vi "amp PID.vi"(0 "D gain":fxp<+/-,32,11>, 1 "Input":i16, 2 "hp coeff":i32[](array[numeric])=[946630756, 1010186290], 7 "I gain":fxp<+/-,32,11>, 8 "Upper limit":fxp<+/-,32,2>, 9 "P gain":fxp<+/-,32,11>, 10 "Lower limit":fxp<+/-,32,2>, 11 "Reset Integral":bool, 12 "DC offset":i16, 13 "lp coeff":i32[](array[numeric])=[1008310688, 32715568], 15 "final filter coeff":i32[](array[numeric])=[-955995012, 2025731616, 1001305, -1023351008, 2092954700, 1034533]) -> (3 "P gain check":fxp<+/-,32,2> format="%.31g", 4 "Final Filter check":fxp<+/-,32,2> format="%.31g", 5 "coerce check":fxp<+/-,32,2> format="%.31g", 6 "PID Output":fxp<+/-,32,2> format="%.26g", 14 "Divide check":fxp<+/-,32,2> format="%.31g")   [LabVIEW 2020]
uses:
  <vilib>/rvi/FXPMathLib/basic elements/FxpIntAccumulator/subVIs/nifxpmath_IntAccumulator_SimConfig.ctl
  <vilib>/rvi/FXPMathLib/basic elements/FxpIntAccumulator/simVIs/DllFxpIntAccumulator_sub.vi
  <vilib>/rvi/Analysis/measure/butterworth/XNode/niFpgaButterworthFilter.xnode
  <vilib>/rvi/FXPMathLib/basic elements/FxpIntAccumulator/XNode/nifxpmath_IntAccumulator.xnode
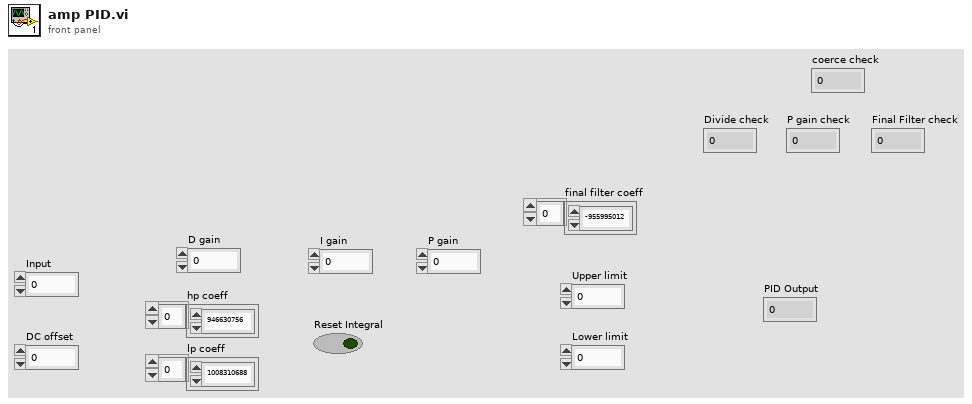
[diagram p1: front panel]
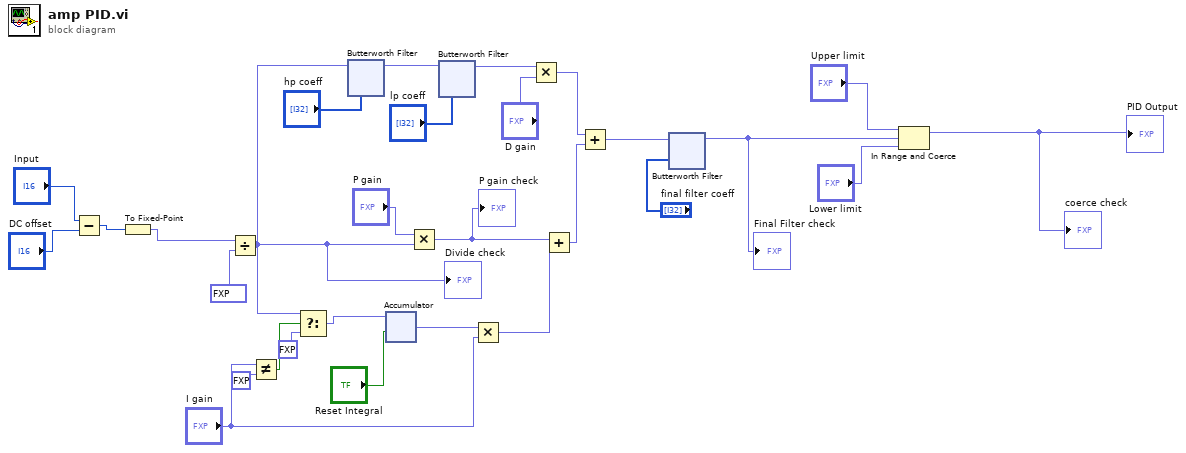
[diagram p0: block diagram]
diagram:
  n1 = Subtract(x="Input", y="DC offset") -> (x-y=w6:i16)
  n2 = To Fixed-Point(number=w6) -> (fixed-point=w5:fxp<+/-,32,16>)  [unwired: 1 in]
  n3 = Divide(x=w5, y=fxp<+,1,15> 16384.0) -> (x/y=w8:fxp<+/-,32,2>)
  "Divide check" <- w8
  n4 = Not Equal?(x="I gain", y=fxp<+/-,16,16> 0.0) -> (x != y?=w20:bool)
  n5 = Select(t=w8, s=w20, f=fxp<+/-,32,2> 0.0) -> (s? t:f=w18:fxp<+/-,32,2>)
  n6 = xnode "Butterworth Filter"("input data"=w8, "scaled coefficients"="hp coeff") -> ("output data"=w13:fxp<+/-,36,6>)  [unwired: 1 in]
  n7 = xnode "Accumulator"("x"=w18, "load (F)"="Reset Integral") -> ("s"=w29:fxp<+/-,46,16>)  [unwired: 3 in, 1 out]
  n8 = Multiply(x="P gain", y=w8) -> (x*y=w7:fxp<+/-,32,2>)
  "P gain check" <- w7
  n9 = xnode "Butterworth Filter"("input data"=w13, "scaled coefficients"="lp coeff") -> ("output data"=w12:fxp<+/-,36,10>)  [unwired: 1 in]
  n10 = Multiply(x=w29, y="I gain") -> (x*y=w26:fxp<+/-,32,2>)
  n11 = Multiply(x=w12, y="D gain") -> (x*y=w17:fxp<+/-,32,2>)
  n12 = Add(x=w7, y=w26) -> (x+y=w25:fxp<+/-,32,2>)
  n13 = Add(x=w17, y=w25) -> (x+y=w14:fxp<+/-,32,2>)
  n14 = xnode "Butterworth Filter"("input data"=w14, "scaled coefficients"="final filter coeff") -> ("output data"=w4:fxp<+/-,32,2>)  [unwired: 1 in]
  "Final Filter check" <- w4
  n15 = In Range and Coerce(upper limit="Upper limit", x=w4, lower limit="Lower limit") -> (coerced(x)=→"PID Output" →"coerce check":fxp<+/-,32,2>)  [unwired: 1 out]
